vi "Read Target Temperature.vi"   [LabVIEW 2013, in "LVH-Nest.lvlib"]
uses:
  LVH-Nest.lvlib
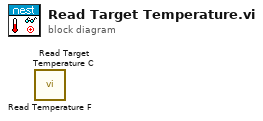
[diagram p0: block diagram]
diagram:
  n1 = call "Read Temperature F.vi"() -> ()  [unwired: 9 in, 3 out]
  n2 = call "Read Target Temperature C.vi"() -> ()  [unwired: 7 in, 5 out]
